vi "ssh2.vi"() -> ()   [LabVIEW 2013]
doc: "This VI illustrates how to connect to a remote SSH server."
uses:
  libssh2/Hostkey Hash Type.ctl
  libssh2/libssh2.lvlib
panel:
  out "exit status":i32
  in  "command":string="echo \"Hello World\""
  out "response":string
  out "supported authentication methods":string
  in  "password":string
  in  "username":string
  out "fingerprint":string
  in  "address":string
  out "error out":errorcluster
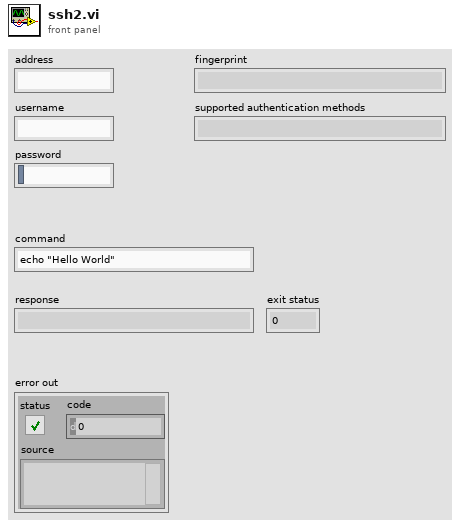
[diagram p1: front panel]
types:
  T1 = typedef "libssh2.lvlib/Hostkey Hash Type.ctl" = enum16{"MD5", "SHA1", "SHA256"}
  T2 = typedef "libssh2.lvlib/Session Refnum.ctl" = refnum<k1>
  T3 = typedef "libssh2.lvlib/Channel Refnum.ctl" = refnum<k1>
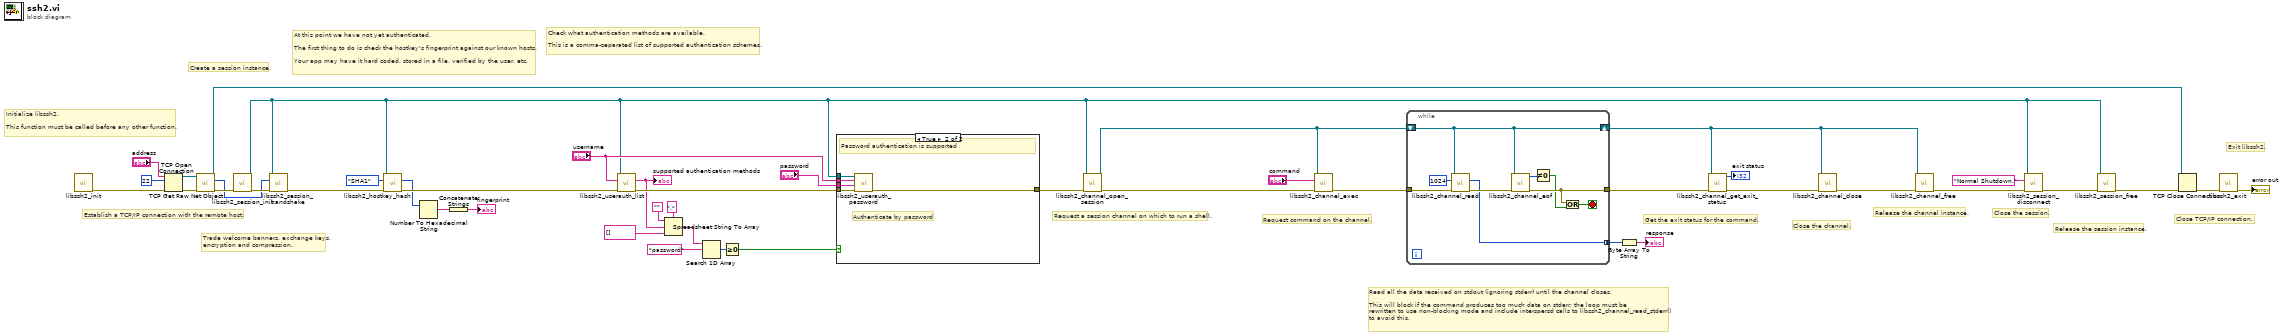
[diagram p0: block diagram]
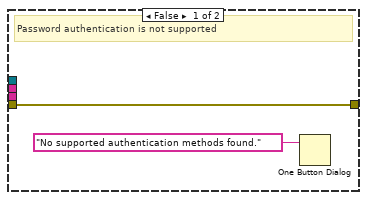
[diagram p2: hidden frame]
diagram:
  # "Close the session."
  # "Close the channel."
  # "Get the exit status for the command."
  # "Read all the data received on stdout (ignoring stderr) until the channel closes.\n\nThis will block if the command produces too much data on stderr; the loop must be\nrewritten to use non-blocking mode and include interspersd calls to libssh2_channel_read_stderr()\nto avoid this."
  # "Release the channel instance."
  # "Request command on the channel."
  # "Request a session channel on which to run a shell."
  # "Check what authentication methods are available.\n\nThis is a comma-separated list of supported authentication schemes."
  # "Close TCP/IP connection."
  # "Exit libssh2."
  # "Release the session instance."
  # "Initialize libssh2.\n\nThis function must be called before any other function."
  # "Establish a TCP/IP connection with the remote host."
  # "At this point we have not yet authenticated.\n\nThe first thing to do is check the hostkey's fingerprint against our known hosts.\n\nYour app may have it hard coded, stored in a file, verified by the user, etc."
  # "Trade welcome banners, exchange keys,\nencryption and compression."
  # "Create a session instance."
  n1 = call "libssh2_init.vi"() -> ("error out"=w45:errorcluster)  [unwired: 10 in, 1 out]
  n2 = TCP Open Connection(address="address", remote port or service name=u16 22, error in (no error)=w45) -> (connection ID=w39:refnum<k5>, error out=w41:errorcluster)  [unwired: 2 in]
  n3 = call <vilib>:"TCP Get Raw Net Object.vi"("error in (no error)"=w41, "connection ID"=w39) -> ("error out"=w40:errorcluster, "raw net object"=w34:u64, "connection ID out"=w37:refnum<k5>)  [unwired: 7 in]
  n4 = call "libssh2_session_init.vi"("error in (no error)"=w40) -> ("error out"=w36:errorcluster, "session"=w1:T2)  [unwired: 9 in]
  n5 = call "libssh2_session_handshake.vi"("error in (no error)"=w36, "socket"=w34, "session"=w1) -> ("error out"=w35:errorcluster)  [unwired: 7 in, 1 out]
  n6 = call "libssh2_hostkey_hash.vi"("error in (no error)"=w35, "hash type"=Hostkey_Hash_Type."SHA1", "session"=w1) -> ("error out"=w33:errorcluster, "hash"=w30:u8[])  [unwired: 7 in]
  n7 = Number To Hexadecimal String(2:w30) -> (0:w29:string[])  [unwired: 1 in]
  n8 = Concatenate Strings(w29) -> (→"fingerprint":string)
  n9 = call "libssh2_userauth_list.vi"("error in (no error)"=w33, "username"="username", "session"=w1) -> ("error out"=w27:errorcluster, "supported authentication schemes"=w26:string)  [unwired: 7 in]
  "supported authentication methods" <- w26
  n10 = Spreadsheet String To Array(delimiter (Tab)=",", format string="", spreadsheet string=w26, array type (2D Dbl)=string[] []) -> (array=w22:string[])
  n11 = Search 1D Array(1D array=w22, element="password") -> (index of element=w17:i32)  [unwired: 1 in]
  n12 = Greater Or Equal To 0?(x=w17) -> (x >= 0?=w16:bool)
  n13 = case shown="True" w16 {
    tunnel: w27 -> [w47 w52]
    tunnel: [w47 w51] -> w20
    tunnel: w1 -> [_ w50]
    tunnel: "username" -> [_ w49]
    tunnel: "password" -> [_ w48]
    frame False {
      # "Password authentication is not supported"
      n14 = One Button Dialog(message="No supported authentication methods found.") -> ()  [unwired: 1 in, 1 out]
    }
    frame True {
      # "Authenticate by password"
      # "Password authentication is supported"
      n15 = call "libssh2_userauth_password.vi"("error in (no error)"=w52, "password"=w48, "username"=w49, "session"=w50) -> ("error out"=w51:errorcluster)  [unwired: 6 in, 1 out]
    }
  }
  n16 = call "libssh2_channel_open_session.vi"("error in (no error)"=w20, "session"=w1) -> ("error out"=w15:errorcluster, "channel"=w10:T3)  [unwired: 8 in]
  n17 = call "libssh2_channel_exec.vi"("error in (no error)"=w15, "command"="command", "channel"=w10) -> ("error out"=w14:errorcluster)  [unwired: 7 in, 1 out]
  n18 = while {
    tunnel: w14 -> [w61]
    tunnel: [w59] -> w11
    shift-right: [w55] -> w4
    shift-left: w10 -> [w55]
    tunnel: [w53] -> w9 mode=concatenating
    stop <- w60 stop-if-true
    n19 = call "libssh2_channel_read.vi"("error in (no error)"=w61, "buflen"=i64 1024, "channel"=w55) -> ("error out"=w56:errorcluster, "buf"=w53:u8[])  [unwired: 6 in, 1 out]
    n20 = call "libssh2_channel_eof.vi"("error in (no error)"=w56, "channel"=w55) -> ("error out"=w59:errorcluster, "return value"=w58:i32)  [unwired: 8 in]
    n21 = Not Equal To 0?(x=w58) -> (x != 0?=w57:bool)
    n22 = Or(x=w59, y=w57) -> (x .or. y?=w60:bool)
  }
  n23 = Byte Array To String(unsigned byte array=w9) -> (string=→"response":string)
  n24 = call "libssh2_channel_get_exit_status.vi"("error in (no error)"=w11, "channel"=w4) -> ("error out"=w7:errorcluster, "return value"=→"exit status":i32)  [unwired: 8 in]
  n25 = call "libssh2_channel_close.vi"("error in (no error)"=w7, "channel"=w4) -> ("error out"=w5:errorcluster)  [unwired: 8 in, 1 out]
  n26 = call "libssh2_channel_free.vi"("error in (no error)"=w5, "channel"=w4) -> ("error out"=w12:errorcluster)  [unwired: 8 in, 1 out]
  n27 = call "libssh2_session_disconnect.vi"("error in (no error)"=w12, "description"="Normal Shutdown.", "session"=w1) -> ("error out"=w3:errorcluster)  [unwired: 7 in, 1 out]
  n28 = call "libssh2_session_free.vi"("error in (no error)"=w3, "session"=w1) -> ("error out"=w31:errorcluster)  [unwired: 8 in, 1 out]
  n29 = TCP Close Connection(connection ID=w37, error in (no error)=w31) -> (error out=w38:errorcluster)  [unwired: 1 in, 1 out]
  n30 = call "libssh2_exit.vi"("error in (no error)"=w38) -> ("error out"=→"error out":errorcluster)  [unwired: 10 in]
